vi "List Keys.vi"(11 "Object Dictionary":refnum<class "objdict.lvclass">) -> (3 "keys":string[](array[string]))   [LabVIEW 2015, in "objdict.lvclass"]
doc: "Lists the keys of all objects in the dictionary."
uses:
  objdict.lvclass
  objdict.lvclass/objdict.ctl
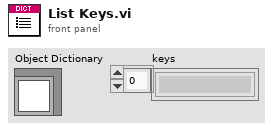
[diagram p1: front panel]
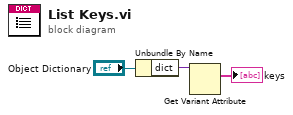
[diagram p0: block diagram]
diagram:
  n1 = Unbundle By Name("Object Dictionary") -> ("dict"=w2:variant)
  n2 = Get Variant Attribute(Variant=w2) -> (names=→"keys":string[])  [unwired: 3 in, 3 out]
